vi "Log_ADAM_scan_table.vi"() -> ()   [LabVIEW 2015]
uses:
  ADAM Client/Sub VIs/ADAM Controls/Channel_State.ctl
  Anemometry/Anemometry Sub Vis/Globals/Constants_global.vi
  Anemometry/Anemometry Sub Vis/Globals/Preference_global.vi
  ADAM_Global.vi
  Anemometry/Anemometry Sub Vis/Globals/Meas_global.vi
panel:
  in  "Ventilate Lab if temp above":dbl=21.5
  in  "Averaging time (Seconds)":dbl=60.0
  out "Current time":string
  out "Started Time":string
  in  "stop":bool
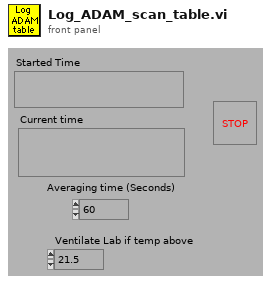
[diagram p1: front panel]
types:
  T1 = enum16{"On", "Off", "Always On", "Always Off", "Delete"}
  T2 = typedef "Channel_State.ctl" = enum16{"On", "Off", "Always On", "Always Off"}
  T3 = enum16{"Load ADAM setup from excel file", "Save ADAM setup to excel file"}
  T4 = cluster{"second":i32, "minute":i32, "hour":i32, "day of month":i32, "month":i32, "year":i32, "day of week":i32, "day of year":i32, "is DST":i32}
  T5 = typedef "Client_State_Cluster.ctl" = cluster{"Client Name":string, "Traverse level State":T6, "People to Email":string[], "Next Contact Time":dbl}
  T6 = typedef "Traverse_Level_State.ctl" = enum16{"Running", "Complete"}
  T7 = typedef "Server_Control.ctl" = cluster{"Channel Name to control":string, "Channel sharing":enum16{"Channel Unshared", "Channel Shared by Rig", "Channel Shared by Group"}, "Default Value":dbl, "Client Array":string[], "Time Stamp":timestamp, "Do Not Reset":bool}
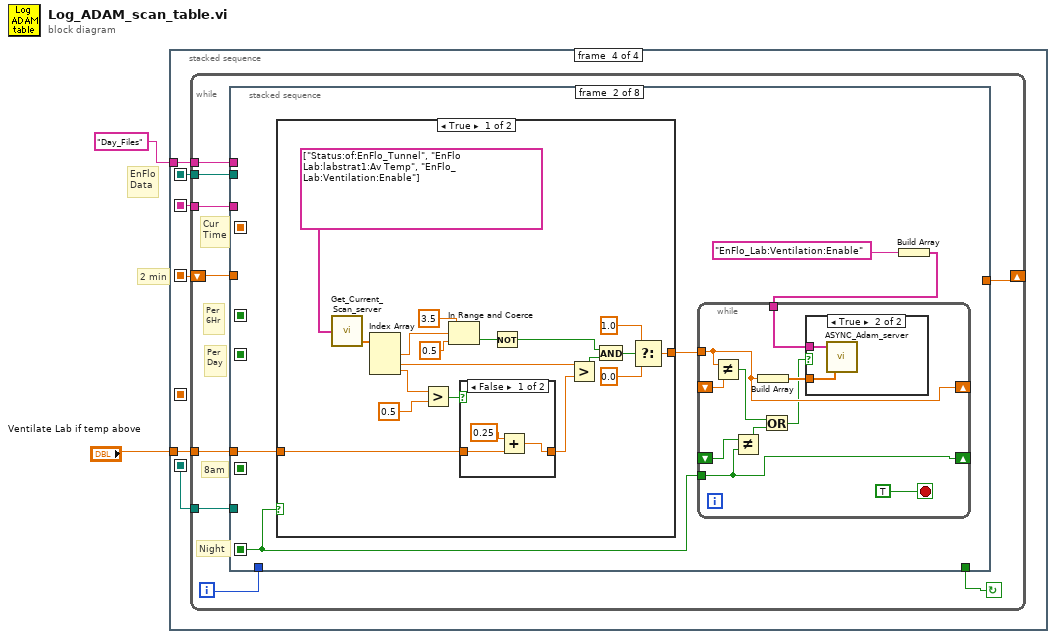
[diagram p0: block diagram]
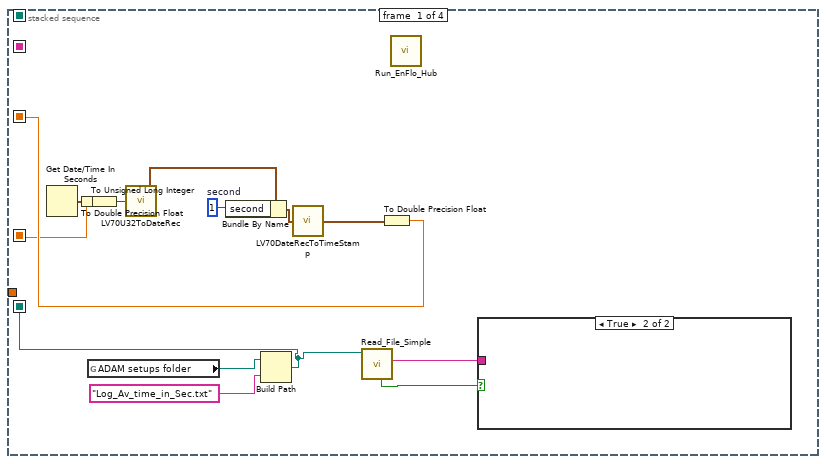
[diagram p2: hidden frame]
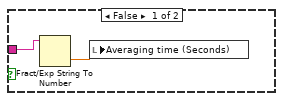
[diagram p3: hidden frame]
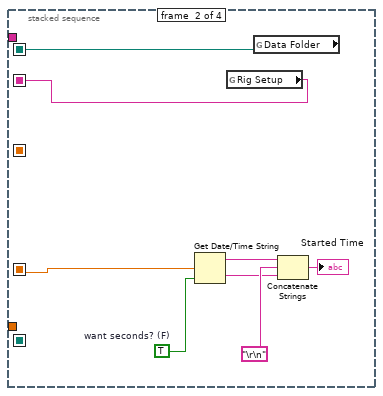
[diagram p4: hidden frame]
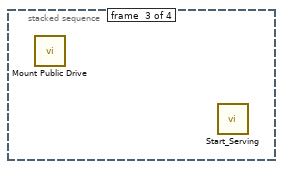
[diagram p5: hidden frame]
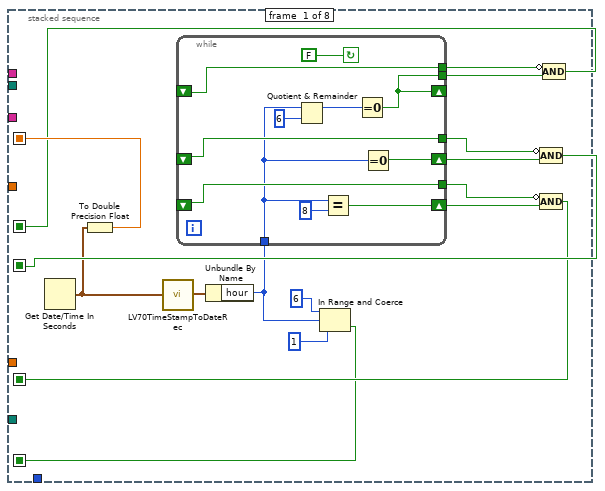
[diagram p6: hidden frame]
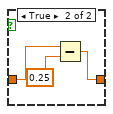
[diagram p8: hidden frame]
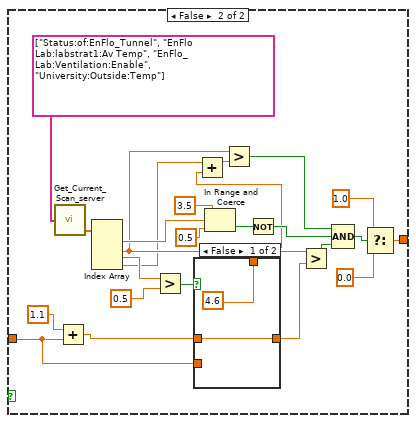
[diagram p9: hidden frame]
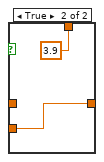
[diagram p10: hidden frame]
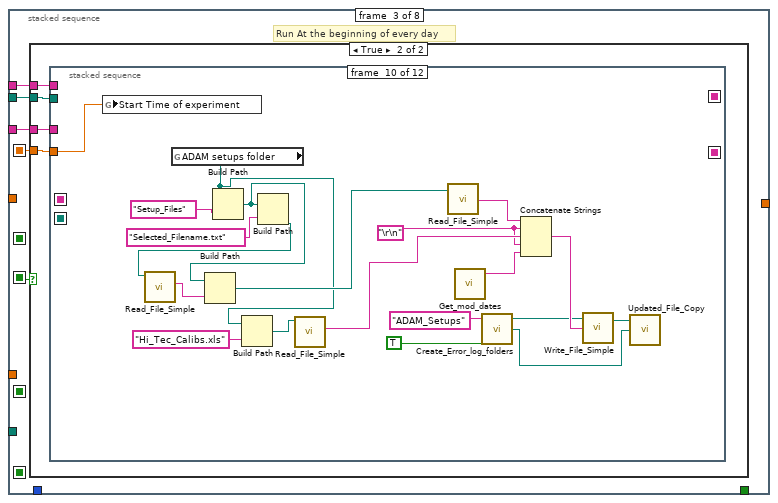
[diagram p11: hidden frame]
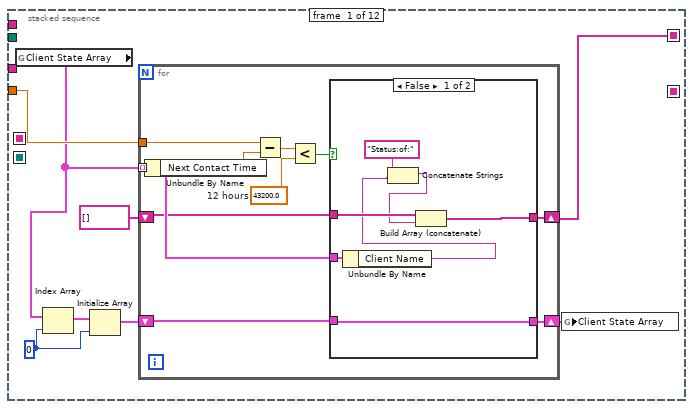
[diagram p13: hidden frame]
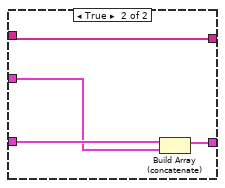
[diagram p14: hidden frame]
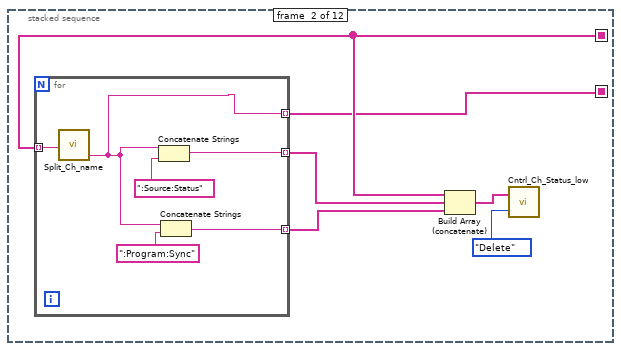
[diagram p15: hidden frame]
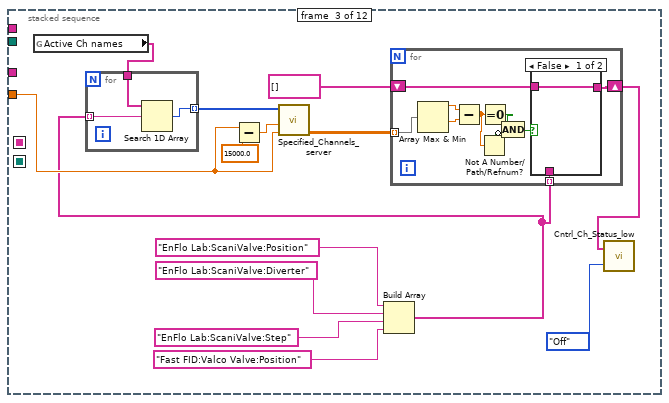
[diagram p16: hidden frame]
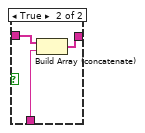
[diagram p17: hidden frame]
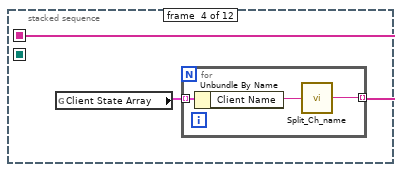
[diagram p18: hidden frame]
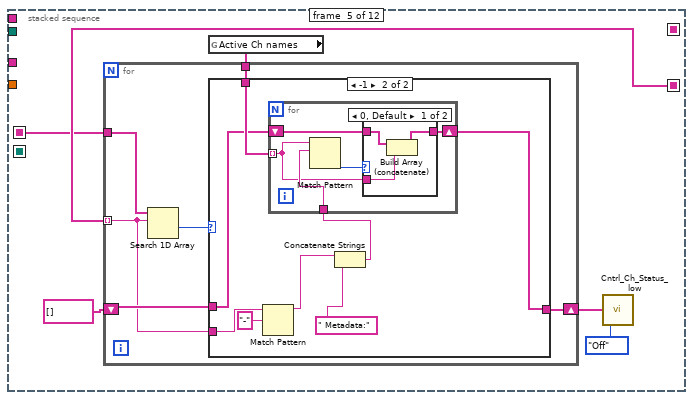
[diagram p19: hidden frame]
diagram:
  # "EnFlo\nData"
  # "2 min"
  n1 = stacked-sequence {
    seq-local: [w13 _ _ _] -> [_ _ _ w31]
    seq-local: [w12 _ _ _] -> [_ w25 _ _]
    seq-local: [_ w19 _ _] -> [_ _ _ w30]
    seq-local: [w5 _ _ _] -> [_ _ _ w28]
    seq-local: [_ w18 _ _] -> [_ _ _ w27]
    tunnel: "Day_Files" ("Input Element") -> [_ _ _ w29]
    tunnel: "Ventilate Lab if temp above" -> [_ _ _ w26]
    frame #0 {
      w15 = 1  # second
      n2 = Get Date/Time In Seconds() -> (seconds since 1Jan1904=w9:timestamp)
      n3 = To Double Precision Float(number=w9) -> (double precision float=w12:dbl)
      n4 = global read "Constants_global.vi" "ADAM setups folder"() -> (w7:path)
      n5 = To Unsigned Long Integer(number=w12) -> (unsigned 32bit integer=w11:u32)
      n6 = call <vilib>:"LV70U32ToDateRec.vi"("Time"=w11) -> ("date time rec"=w10:T4)
      n7 = Bundle By Name(cluster=w10, "second"=w15) -> (w14:T4)
      n8 = Build Path(base path=w7, name or relative path="Log_Av_time_in_Sec.txt") -> (appended path=w5:path)
      n9 = call <vilib>:"LV70DateRecToTimeStamp.vi"("date time rec"=w14) -> ("Time Stamp"=w8:timestamp)
      n10 = call "Read_File_Simple.vi"("Filename"=w5) -> ("Error?"=w3:bool, "string"=w4:string)  [unwired: 2 in, 6 out]
      n11 = To Double Precision Float(number=w8) -> (double precision float=w13:dbl)
      n12 = call "Run_EnFlo_Hub.vi"() -> ()  [unwired: 8 out]
      n13 = case shown="True" w3 {
        tunnel: w4 -> [w17 _]
        frame False {
          n14 = Fract/Exp String To Number(string=w17) -> (number=w16:dbl)  [unwired: 4 out]
          n15 = local write "Averaging time (Seconds)"(w16) -> ()
        }
        frame True {
        }
      }
    }
    frame #1 {
      w24 = TRUE  # want seconds? (F)
      n16 = Get Date/Time String(seconds (now)=w25, want seconds? (F)=w24) -> (date string=w22:string, time string=w21:string)  [unwired: 1 out]
      n17 = global read "Preference_global.vi" "Rig Setup"() -> (w18:string)
      n18 = global read "Constants_global.vi" "Data Folder"() -> (w19:path)
      n19 = Concatenate Strings(w22, "\r\n", w21) -> (→"Started Time":string)
    }
    frame #2 {
      n20 = call "Mount Public Drive.vi"() -> ()  [unwired: 12 in]
      n21 = call "Start_Serving.vi"() -> ()  [unwired: 1 out]
    }
    frame #3 {
      n22 = while {
        tunnel: w30 -> [w38]
        shift-left: w31 -> [w40]
        shift-right: [w39] -> _
        tunnel: w29 -> [w35]
        tunnel: w28 -> [w34]
        tunnel: w27 -> [w33]
        tunnel: w26 -> [w32]
        i -> [w37]
        stop <- w36 continue-if-true
        # "Night"
        # "8am"
        # "Per\n6Hr"
        # "Per\nDay"
        # "Cur\nTime"
        n23 = stacked-sequence {
          seq-local: [w49 _ _ _ _ _ _ _] -> [_ _ w141 _ _ _ _ _]
          seq-local: [w55 _ _ _ _ _ _ _] -> [_ _ w140 w367 w386 _ _ _]
          seq-local: [w52 _ _ _ _ _ _ _] -> [_ _ _ _ _ _ _ _]
          seq-local: [w45 _ _ _ _ _ _ _] -> [_ _ _ w363 _ _ _ _]
          seq-local: [w41 _ _ _ _ _ _ _] -> [_ w68 _ _ _ _ _ _]
          tunnel: [_ _ _ _ _ w388 _ _] -> w39
          tunnel: w40 -> [_ _ _ _ _ w389 _ _]
          tunnel: w38 -> [_ _ w139 w366 _ w396 _ _]
          tunnel: w37 -> [_ _ _ _ _ _ _ _]
          tunnel: [_ _ _ _ _ _ _ w428] -> w36
          tunnel: w35 -> [_ _ w138 w365 _ w397 _ _]
          tunnel: w34 -> [_ _ _ _ _ _ _ w427]
          tunnel: w33 -> [_ _ w137 w364 _ w390 _ _]
          tunnel: w32 -> [_ w69 _ _ _ _ _ _]
          frame #0 {
            n24 = Get Date/Time In Seconds() -> (seconds since 1Jan1904=w48:timestamp)
            n25 = To Double Precision Float(number=w48) -> (double precision float=w55:dbl)
            n26 = call <vilib>:"LV70TimeStampToDateRec.vi"("time stamp"=w48) -> ("date time rec"=w56:T4)
            n27 = Unbundle By Name(w56) -> ("hour"=w44:i32)
            n28 = while {
              tunnel: [w62] -> w50
              shift-left: _ -> [w62]
              shift-right: [w63] -> w51
              tunnel: [w64] -> w53
              tunnel: [w65] -> w54
              tunnel: w44 -> [w59]
              shift-left: _ -> [w64]
              shift-right: [w65] -> _
              tunnel: [w60] -> w47
              shift-right: [w57] -> w46
              shift-left: _ -> [w60]
              stop <- FALSE continue-if-true
              n29 = Quotient & Remainder(x=w59, y=6) -> (x-y*floor(x/y)=w66:i32)  [unwired: 1 out]
              n30 = Equal?(x=w59, y=8) -> (x = y?=w57:bool)
              n31 = Equal To 0?(x=w66) -> (x = 0?=w65:bool)
              n32 = Equal To 0?(x=w59) -> (x = 0?=w63:bool)
            }
            n33 = In Range and Coerce(upper limit=6, x=w44, lower limit=1) -> (In Range?=w41:bool)  [unwired: 1 out]
            n34 = Compound Arithmetic op=AND(invert w50, w51) -> (w49:bool)
            n35 = Compound Arithmetic op=AND(invert w47, w46) -> (w45:bool)
            n36 = Compound Arithmetic op=AND(invert w53, w54) -> (w52:bool)
          }
          frame #1 {
            n37 = case shown="True" w68 {
              tunnel: [w95 w126] -> w70
              tunnel: w69 -> [w85 w109]
              frame True {
                n38 = call "Get_Current_Scan_server.vi"("Desired Channels"=string[] ["Status:of:EnFlo_Tunnel", "EnFlo Lab:labstrat1:Av Temp", "EnFlo_Lab:Ventilation:Enable"]) -> ("Numerical Values"=w101:dbl[])  [unwired: 2 out]
                n39 = Index Array(array=w101) -> (element #1=w94:dbl, element #2=w100:dbl, element #3=w89:dbl)  [unwired: 3 in]
                n40 = Greater?(x=w89, y=0.5) -> (0:w87:bool)
                n41 = In Range and Coerce(upper limit=3.5, x=w94, lower limit=0.5) -> (In Range?=w91:bool)  [unwired: 1 out]
                n42 = case shown="False" w87 {
                  tunnel: [w104 w106] -> w86
                  tunnel: w85 -> [w105 w108]
                  frame False {
                    n43 = Add(x=0.25, y=w105) -> (x+y=w104:dbl)
                  }
                  frame True {
                    n44 = Subtract(x=w108, y=0.25) -> (x-y=w106:dbl)
                  }
                }
                n45 = Not(x=w91) -> (.not. x?=w90:bool)
                n46 = Greater?(x=w100, y=w86) -> (0:w99:bool)
                n47 = And(x=w90, y=w99) -> (x .and. y?=w98:bool)
                n48 = Select(t=1.0, s=w98, f=0.0) -> (s? t:f=w95:dbl)
              }
              frame False {
                n49 = call "Get_Current_Scan_server.vi"("Desired Channels"=string[] ["Status:of:EnFlo_Tunnel", "EnFlo Lab:labstrat1:Av Temp", "EnFlo_Lab:Ventilation:Enable", "University:Outside:Temp"]) -> ("Numerical Values"=w131:dbl[])  [unwired: 2 out]
                n50 = Add(x=1.1, y=w109) -> (x+y=w116:dbl)
                n51 = Index Array(array=w131) -> (element #1=w125:dbl, element #2=w114:dbl, element #3=w120:dbl, element #4=w113:dbl)  [unwired: 4 in]
                n52 = Greater?(x=w120, y=0.5) -> (0:w118:bool)
                n53 = case shown="False" w118 {
                  tunnel: [w134 w135] -> w117
                  tunnel: w116 -> [w134 _]
                  tunnel: [4.6 ("y") 3.9 ("y")] -> w110
                  tunnel: w109 -> [_ w135]
                  frame False {
                  }
                  frame True {
                  }
                }
                n54 = Add(x=w113, y=w110) -> (x+y=w112:dbl)
                n55 = In Range and Coerce(upper limit=3.5, x=w125, lower limit=0.5) -> (In Range?=w122:bool)  [unwired: 1 out]
                n56 = Greater?(x=w114, y=w112) -> (0:w111:bool)
                n57 = Not(x=w122) -> (.not. x?=w121:bool)
                n58 = Greater?(x=w114, y=w117) -> (0:w130:bool)
                n59 = Compound Arithmetic op=AND(w111, w121, w130) -> (w129:bool)
                n60 = Select(t=1.0, s=w129, f=0.0) -> (s? t:f=w126:dbl)
              }
            }
            n61 = Build Array("EnFlo_Lab:Ventilation:Enable") -> (w71:string[])
            n62 = while {
              shift-right: [w80] -> _
              shift-left: _ -> [w81]
              tunnel: w70 -> [w80]
              tunnel: w71 -> [w78]
              shift-right: [w77] -> _
              shift-left: _ -> [w76]
              tunnel: w68 -> [w77]
              stop <- TRUE stop-if-true
              n63 = Not Equal?(x=w80, y=w81) -> (x != y?=w74:bool)
              n64 = Not Equal?(x=w76, y=w77) -> (x != y?=w75:bool)
              n65 = Build Array(w80) -> (w82:dbl[])
              n66 = Or(x=w74, y=w75) -> (x .or. y?=w73:bool)
              n67 = case shown="True" w73 {
                tunnel: w82 -> [_ w84]
                tunnel: w78 -> [_ w83]
                frame False {
                }
                frame True {
                  n68 = call "ASYNC_Adam_server.vi"("Values"=w84, "Channel Names"=w83) -> ()  [unwired: 1 in, 3 out]
                }
              }
            }
          }
          frame #2 {
            # "Run At the beginning of every day"
            n69 = case shown="True" w141 {
              tunnel: w140 -> [_ w145]
              tunnel: w139 -> [_ w144]
              tunnel: w138 -> [_ w143]
              tunnel: w137 -> [_ w142]
              frame False {
              }
              frame True {
                n70 = stacked-sequence {
                  seq-local: [w146 _ _ _ _ _ _ _ _ _ _ _] -> [_ w180 _ _ _ _ _ _ w300 _ _ _]
                  seq-local: [_ w176 _ _ _ _ _ _ _ _ _ _] -> [_ _ _ _ w228 _ _ _ _ _ _ _]
                  seq-local: [_ _ _ w218 _ _ _ _ _ _ _ _] -> [_ _ _ _ w225 _ _ _ _ _ _ _]
                  seq-local: [_ _ _ _ _ _ _ _ _ _ w349 _] -> [_ _ _ _ _ _ _ _ _ _ _ w353]
                  tunnel: w145 -> [w153 _ w197 _ _ _ _ _ _ w347 _ w354]
                  tunnel: w144 -> [_ _ _ _ _ _ _ _ _ _ _ _]
                  tunnel: w143 -> [_ _ _ _ _ _ _ _ _ _ _ _]
                  tunnel: w142 -> [_ _ _ _ _ _ _ _ _ _ _ _]
                  frame #0 {
                    w151 = 0 ("Index")
                    n71 = global read "ADAM_Global.vi" "Client State Array"() -> (w152:T5[])
                    n72 = Index Array(array=w152, index=w151) -> (element=w150:T5)
                    n73 = Initialize Array(w150, w151) -> (w149:T5[])
                    n74 = for {
                      tunnel: w152 -> [w156] mode=indexing
                      shift-right: [w157] -> w148
                      shift-left: w149 -> [w158]
                      tunnel: w153 -> [w163]
                      shift-right: [w154] -> w146
                      shift-left: string[] [] -> [w155]
                      w160 = 43200.0  # 12 hours
                      n75 = Unbundle By Name(w156) -> ("Next Contact Time"=w162:dbl)
                      n76 = Subtract(x=w163, y=w162) -> (x-y=w161:dbl)
                      n77 = Less?(x=w161, y=w160) -> (x < y?=w159:bool)
                      n78 = case shown="False" w159 {
                        tunnel: w158 -> [w170 w174]
                        tunnel: [w170 w173] -> w157
                        tunnel: w156 -> [w169 w172]
                        tunnel: w155 -> [w168 w171]
                        tunnel: [w167 w171] -> w154
                        frame False {
                          n79 = Unbundle By Name(w169) -> ("Client Name"=w165:string)
                          n80 = Concatenate Strings("Status:of:", w165) -> (w164:string)
                          n81 = Build Array (concatenate)(w168, w164) -> (w167:string[])
                        }
                        frame True {
                          n82 = Build Array (concatenate)(w174, w172) -> (w173:T5[])
                        }
                      }
                    }
                    n83 = global write "ADAM_Global.vi" "Client State Array"(w148) -> ()
                  }
                  frame #1 {
                    n84 = for {
                      tunnel: w180 -> [w186] mode=indexing
                      tunnel: [w183] -> w178 mode=indexing
                      tunnel: [w182] -> w177 mode=indexing
                      tunnel: [w181] -> w176 mode=indexing
                      n85 = call "Split_Ch_name.vi"("Ch name"=w186) -> ("Low level"=w181:string)  [unwired: 2 out]
                      n86 = Concatenate Strings(w181, ":Source:Status") -> (w183:string)
                      n87 = Concatenate Strings(w181, ":Program:Sync") -> (w182:string)
                    }
                    n88 = Build Array (concatenate)(w180, w178, w177) -> (w179:string[])
                    n89 = call "Cntrl_Ch_Status_low.vi"("Mode"=T1."Delete", "Channel names"=w179) -> ()  [unwired: 1 out]
                  }
                  frame #2 {
                    n90 = global read "ADAM_Global.vi" "Active Ch names"() -> (w200:string[])
                    n91 = Subtract(x=w197, y=15000.0) -> (x-y=w195:dbl)
                    n92 = Build Array("EnFlo Lab:ScaniValve:Position", "EnFlo Lab:ScaniValve:Diverter", "EnFlo Lab:ScaniValve:Step", "Fast FID:Valco Valve:Position") -> (w193:string[])
                    n93 = for {
                      tunnel: w200 -> [w217]
                      tunnel: w193 -> [w216] mode=indexing
                      tunnel: [w215] -> w198 mode=indexing
                      n94 = Search 1D Array(1D array=w217, element=w216) -> (index of element=w215:i32)  [unwired: 1 out]
                    }
                    n95 = call "Specified_Channels_server.vi"("End time"=w197, "Start time"=w195, "Requested channels"=w198) -> ("Output array"=w194:dbl[][])  [unwired: 2 in, 4 out]
                    n96 = for {
                      tunnel: w194 -> [w207] mode=indexing
                      shift-right: [w208] -> w188
                      shift-left: string[] [] -> [w202]
                      tunnel: w193 -> [w203] mode=indexing
                      n97 = Array Max & Min(array=w207) -> (max value=w210:dbl, min value=w209:dbl)  [unwired: 2 out]
                      n98 = Subtract(x=w210, y=w209) -> (x-y=w206:dbl)
                      n99 = Not A Number/Path/Refnum?(number/path/refnum=w206) -> (NaN/Path/Refnum?=w204:bool)
                      n100 = Equal To 0?(x=w206) -> (x = 0?=w201:bool)
                      n101 = Compound Arithmetic op=AND(w201, invert w204) -> (w205:bool)
                      n102 = case shown="False" w205 {
                        tunnel: [w211 w214] -> w208
                        tunnel: w203 -> [_ w213]
                        tunnel: w202 -> [w211 w212]
                        frame False {
                        }
                        frame True {
                          n103 = Build Array (concatenate)(w212, w213) -> (w214:string[])
                        }
                      }
                    }
                    n104 = call "Cntrl_Ch_Status_low.vi"("Mode"=T1."Off", "Channel names"=w188) -> ()  [unwired: 1 out]
                  }
                  frame #3 {
                    n105 = global read "ADAM_Global.vi" "Client State Array"() -> (w219:T5[])
                    n106 = for {
                      tunnel: w219 -> [w222] mode=indexing
                      tunnel: [w220] -> w218 mode=indexing
                      n107 = Unbundle By Name(w222) -> ("Client Name"=w221:string)
                      n108 = call "Split_Ch_name.vi"("Ch name"=w221) -> ("Middle"=w220:string)  [unwired: 2 out]
                    }
                  }
                  frame #4 {
                    n109 = global read "ADAM_Global.vi" "Active Ch names"() -> (w226:string[])
                    n110 = for {
                      tunnel: w228 -> [w229] mode=indexing
                      shift-right: [w232] -> w224
                      shift-left: string[] [] -> [w233]
                      tunnel: w226 -> [w231]
                      tunnel: w225 -> [w230]
                      n111 = Search 1D Array(1D array=w230, element=w229) -> (index of element=w234:i32)  [unwired: 1 out]
                      n112 = case shown="-1" w234 {
                        tunnel: w233 -> [w235 w241]
                        tunnel: [w235 w240] -> w232
                        tunnel: w229 -> [_ w236]
                        tunnel: w231 -> [_ w242]
                        frame 0, Default {
                        }
                        frame -1 {
                          n113 = Match Pattern(string=w236, regular expression="-") -> (before substring=w237:string)  [unwired: 4 out]
                          n114 = Concatenate Strings(w237, " Metadata:" ("Substring")) -> (w239:string)
                          n115 = for {
                            shift-right: [w246] -> w240
                            shift-left: w241 -> [w247]
                            tunnel: w239 -> [w245]
                            tunnel: w242 -> [w244] mode=indexing
                            n116 = Match Pattern(string=w244, regular expression=w245) -> (offset past match=w248:i32)  [unwired: 4 out]
                            n117 = case shown="0, Default" w248 {
                              tunnel: w247 -> [w250 w252]
                              tunnel: [w249 w252] -> w246
                              tunnel: w244 -> [w251 _]
                              frame 0, Default {
                                n118 = Build Array (concatenate)(w250, w251) -> (w249:string[])
                              }
                              frame -1 {
                              }
                            }
                          }
                        }
                      }
                    }
                    n119 = call "Cntrl_Ch_Status_low.vi"("Mode"=T1."Off", "Channel names"=w224) -> ()  [unwired: 1 out]
                  }
                  frame #5 {
                    n120 = Build Array("EnFlo_Tunnel:Heater:Enable") -> (w258:string[])
                    n121 = call "Get_Current_Scan_server.vi"("Desired Channels"=w258) -> ("Numerical Values"=w257:dbl[])  [unwired: 2 out]
                    n122 = Index Array(array=w257, index=0) -> (element=w255:dbl)
                    n123 = Less?(x=w255, y=0.5) -> (x < y?=w253:bool)
                    n124 = case shown="True" w253 {
                      frame False {
                      }
                      frame True {
                        w264 = "EnFlo_Tunnel:Setpo"
                        n125 = global read "ADAM_Global.vi" "Active Ch names"() -> (w262:string[])
                        n126 = String Length(string=w264) -> (length=w263:i32)
                        n127 = for {
                          shift-right: [w272] -> w261
                          shift-left: string[] [] -> [w274]
                          tunnel: w262 -> [w273] mode=indexing
                          tunnel: w263 -> [w276]
                          tunnel: w264 -> [w275]
                          tunnel: "EnFlo_Tunnel:Power" -> [w270]
                          n128 = String Subset(string=w273, length (rest)=w276) -> (substring=w271:string)  [unwired: 1 out]
                          n129 = Equal?(x=w271, y=w275) -> (x = y?=w268:bool)
                          n130 = Equal?(x=w271, y=w270) -> (x = y?=w269:bool)
                          n131 = Or(x=w268, y=w269) -> (x .or. y?=w267:bool)
                          n132 = case shown="True" w267 {
                            tunnel: w274 -> [w277 w280]
                            tunnel: w273 -> [_ w279]
                            tunnel: [w277 w278] -> w272
                            frame False {
                            }
                            frame True {
                              n133 = Build Array (concatenate)(w280, w279) -> (w278:string[])
                            }
                          }
                        }
                        n134 = call "Adam_Ch_on_off.vi"("Ch State"=Channel_State."Off", "ADAM Ch Names"=w261) -> ()  [unwired: 1 out]
                      }
                    }
                  }
                  frame #6 {
                    n135 = call "Read_Write_ADAM_setup.vi"("Mode"=T3."Save ADAM setup to excel file") -> ()  [unwired: 4 out]
                  }
                  frame #7 {
                    w285 = 5400.0  # 1.5 Hrs in seconds
                    n136 = Build Array("GMU:Source:Meas Q", "GMU:Source:Est Time") -> (w292:string[])
                    n137 = call "Get_Current_Scan_server.vi"("Desired Channels"=w292) -> ("Numerical Values"=w287:dbl[])  [unwired: 2 out]
                    n138 = Index Array(array=w287, index=0 ("Index")) -> (element=w289:dbl)
                    n139 = Index Array(array=w287, index=1 ("Index")) -> (element=w286:dbl)
                    n140 = Less?(x=w289, y=0.01) -> (x < y?=w283:bool)
                    n141 = Greater?(x=w286, y=w285) -> (0:w284:bool)
                    n142 = And(x=w283, y=w284) -> (x .and. y?=w282:bool)
                    n143 = case shown="True" w282 {
                      frame False {
                      }
                      frame True {
                        w295 = FALSE  # Activate channels
                        w296 = enum16{"Channel Name", "Main Address"}."Channel Name" ("Control on")
                        n144 = call "Ch_Active_Control.vi"("Match"="GMU:", "Activate Channels?"=w295, "Control on"=w296) -> ()  [unwired: 1 in, 2 out]
                        n145 = call "Ch_Active_Control.vi"("Match"="source", "Activate Channels?"=w295, "Control on"=w296) -> ()  [unwired: 1 in, 2 out]
                      }
                    }
                  }
                  frame #8 {
                    w304 = 0 ("Index")
                    n146 = global read "ADAM_Global.vi" "Server Control Array"() -> (w301:T7[])
                    n147 = Index Array(array=w301, index=w304) -> (element=w303:T7)
                    n148 = Initialize Array(w303, w304) -> (w302:T7[])
                    n149 = for {
                      tunnel: w301 -> [w306] mode=indexing
                      shift-right: [w311] -> w299
                      shift-left: w302 -> [w312]
                      tunnel: w300 -> [w310]
                      n150 = Unbundle By Name(w306) -> ("Client Array"=w309:string[])
                      n151 = for {
                        tunnel: w310 -> [w317]
                        tunnel: w309 -> [w315] mode=indexing
                        shift-right: [w313] -> w305
                        shift-left: string[] [] -> [w314]
                        n152 = Search 1D Array(1D array=w317, element=w315) -> (index of element=w316:i32)  [unwired: 1 out]
                        n153 = case shown="0, Default" w316 {
                          tunnel: w315 -> [_ w321]
                          tunnel: w314 -> [w318 w320]
                          tunnel: [w318 w319] -> w313
                          frame 0, Default {
                          }
                          frame -1 {
                            n154 = Build Array (concatenate)(w320, w321) -> (w319:string[])
                          }
                        }
                      }
                      n155 = Array Size(array=w305) -> (size(s)=w307:i32)
                      n156 = case shown="0" w307 {
                        tunnel: w312 -> [w322 w326]
                        tunnel: [w322 w327] -> w311
                        tunnel: w306 -> [_ w325]
                        tunnel: w305 -> [_ w324]
                        frame 0 {
                        }
                        frame 1, Default {
                          n157 = Bundle By Name(cluster=w325, "Client Array"=w324) -> (w323:T7)
                          n158 = Build Array (concatenate)(w326, w323) -> (w327:T7[])
                        }
                      }
                    }
                    n159 = global write "ADAM_Global.vi" "Server Control Array"(w299) -> ()
                  }
                  frame #9 {
                    w335 = "\r\n"
                    n160 = global write "Meas_global.vi" "Start Time of experiment"(w347) -> ()
                    n161 = global read "Constants_global.vi" "ADAM setups folder"() -> (w338:path)
                    n162 = Build Path(base path=w338, name or relative path="Setup_Files") -> (appended path=w342:path)
                    n163 = Build Path(base path=w338, name or relative path="Hi_Tec_Calibs.xls") -> (appended path=w337:path)
                    n164 = Build Path(base path=w342, name or relative path="Selected_Filename.txt" ("Substring")) -> (appended path=w344:path)
                    n165 = call "Read_File_Simple.vi"("Filename"=w344) -> ("string"=w343:string)  [unwired: 2 in, 7 out]
                    n166 = Build Path(base path=w342, name or relative path=w343) -> (appended path=w341:path)
                    n167 = call "Read_File_Simple.vi"("Filename"=w337) -> ("string"=w336:string)  [unwired: 2 in, 7 out]
                    n168 = call "Read_File_Simple.vi"("Filename"=w341) -> ("string"=w340:string)  [unwired: 2 in, 7 out]
                    n169 = call "Get_mod_dates.vi"() -> ("Output string"=w334:string)  [unwired: 1 in, 4 out]
                    n170 = call "Create_Error_log_folders.vi"("Per Day Log File?"=TRUE, "Log Filename"="ADAM_Setups" ("Substring")) -> ("Server copy Location"=w328:path, "Local Log File"=w330:path)  [unwired: 1 in, 1 out]
                    n171 = Concatenate Strings(w340, w335, w336, w335, w334) -> (w331:string)
                    n172 = call "Write_File_Simple.vi"("character string"=w331, "file path"=w330) -> ("file path Out"=w329:path)  [unwired: 1 in, 1 out]
                    n173 = call "Updated_File_Copy.vi"("Target Path"=w328, "Source Path"=w329) -> ()  [unwired: 2 out]
                  }
                  frame #10 {
                    n174 = global read "Constants_global.vi" "Data Folder Local"() -> (w350:path)
                    n175 = Build Path(base path=w350, name or relative path="Results_Summary_files") -> (appended path=w349:path)
                  }
                  frame #11 {
                    # "If the summary files are more than 60 days old delete them"
                    n176 = To Unsigned Long Integer(number=w354) -> (unsigned 32bit integer=w351:u32)
                    n177 = call "Get_folder_and_filenames.vi"("file path (dialog if empty)"=w353) -> ("Files"=w352:path[])  [unwired: 1 out]
                    n178 = for {
                      tunnel: w352 -> [w356] mode=indexing
                      tunnel: w351 -> [w361]
                      # "60 days in seconds"
                      n179 = File/Directory Info(path=w356) -> (last mod=w355:timestamp)  [unwired: 1 in, 6 out]
                      n180 = To Unsigned Long Integer(number=w355) -> (unsigned 32bit integer=w360:u32)
                      n181 = Subtract(x=w361, y=w360) -> (x-y=w359:u32)
                      n182 = Greater?(x=w359, y=u32 5184000) -> (0:w357:bool)
                      n183 = case shown="False" w357 {
                        tunnel: w356 -> [_ w362]
                        frame False {
                        }
                        frame True {
                          n184 = Delete(path (use dialog)=w362) -> ()  [unwired: 1 in, 6 out]
                        }
                      }
                    }
                  }
                }
              }
            }
          }
          frame #3 {
            # "At 8am every day"
            n185 = case shown="True" w363 {
              tunnel: w367 -> [_ w371]
              tunnel: w366 -> [_ w370]
              tunnel: w365 -> [_ w369]
              tunnel: w364 -> [_ w368]
              frame False {
              }
              frame True {
                n186 = stacked-sequence {
                  seq-local: [w379 _] -> [_ w385]
                  tunnel: w371 -> [w383 _]
                  tunnel: w370 -> [w372 _]
                  tunnel: w369 -> [w377 _]
                  tunnel: w368 -> [w373 _]
                  frame #0 {
                    n187 = Subtract(x=w383, y=36000.0) -> (x-y=w381:dbl)
                    n188 = call "Sec_to_date_filename.vi"("seconds"=w381) -> ("Year"=w378:string, "Month"=w382:string, "Day"=w375:string)  [unwired: 1 out]
                    n189 = Concatenate Strings(w375, ".xls" ("string")) -> (w374:string)
                    n190 = Build Array(w378, w373, w377, w382, w374) -> (w380:string[])
                    n191 = call "Build_Pathname.vi"("PathElements"=w380, "PathnameIn"=w372) -> ("AppendedPath"=w379:path)
                  }
                  frame #1 {
                    # "This VI emails a summary of all the server errors that occured Yesterday"
                    n192 = call "Adam_server_messages.vi"("Filename"=w385) -> ()  [unwired: 1 out]
                  }
                }
              }
            }
          }
          frame #4 {
            n193 = call "EnFlo_Seeder_Control.vi"("Current Time (s)"=w386) -> ()
            n194 = Wait (ms)(milliseconds to wait=u32 1000 ("milliseconds to Wait")) -> ()  [unwired: 1 out]
          }
          frame #5 {
            n195 = Divide(x="Averaging time (Seconds)", y=60.0) -> (x/y=w394:dbl)
            n196 = Divide(x="Averaging time (Seconds)", y=2.0) -> (x/y=w391:dbl)
            n197 = Add(x=w391, y=w389) -> (x+y=w407:dbl)
            n198 = call "Sec_to_date_filename.vi"("seconds"=w407) -> ("Year"=w402:string, "Month"=w403:string, "Day"=w398:string)  [unwired: 1 out]
            n199 = Concatenate Strings(w398, ".xls" ("string")) -> (w400:string)
            n200 = Build Array(w402, w390, w397, w403, w400) -> (w401:string[])
            n201 = call "Time_elapsed.vi"("End of previous average in"=w389, "Averaging time (mins)"=w394) -> ("End of previous average out"=w388:dbl, "End of period"=w405:dbl, "Start of period"=w406:dbl, "Time elapsed ?"=w404:bool)  [unwired: 2 in]
            n202 = case shown="True" w404 {
              tunnel: w405 -> [_ w410]
              tunnel: w406 -> [_ w411]
              tunnel: w396 -> [_ w409]
              tunnel: w401 -> [_ w408]
              frame False {
              }
              frame True {
                n203 = stacked-sequence {
                  tunnel: w411 -> [w420 _]
                  tunnel: w410 -> [w419 _]
                  tunnel: w409 -> [w412 _]
                  tunnel: w408 -> [w415 _]
                  frame #0 {
                    n204 = global read "ADAM_Global.vi" "2 Min average comment"() -> (w418:string)
                    n205 = global read "Meas_global.vi" "Error Messages"() -> (w417:string)
                    n206 = call "Build_Pathname.vi"("PathElements"=w415, "PathnameIn"=w412) -> ("AppendedPath"=w414:path)
                    n207 = call "Create_directory_path.vi"("Path name"=w414) -> ("Path name Out"=w413:path)  [unwired: 1 in, 1 out]
                    n208 = Concatenate Strings(w418, w417) -> (w416:string)
                    n209 = call "Write_to_log_file.vi"("User added comment"=w416, "End time"=w419, "Start time"=w420, "Folder/file"=w413) -> ()  [unwired: 5 in, 3 out]
                  }
                  frame #1 {
                    w421 = ""
                    n210 = global write "ADAM_Global.vi" "2 Min average comment"(w421) -> ()
                    n211 = global write "Meas_global.vi" "Error Messages"(w421) -> ()
                  }
                }
              }
            }
          }
          frame #6 {
            w426 = TRUE  # want seconds? (F)
            n212 = Get Date/Time String(want seconds? (F)=w426) -> (date string=w424:string, time string=w423:string)  [unwired: 2 out]
            n213 = Concatenate Strings(w424, "\r\n", w423) -> (→"Current time":string)
          }
          frame #7 {
            n214 = while {
              shift-right: [w430] -> _
              shift-left: _ -> [w434]
              tunnel: w427 -> [w431]
              stop <- TRUE stop-if-true
              n215 = local read "Averaging time (Seconds)"() -> (w430:dbl)
              n216 = Not Equal?(x=w430, y=w434) -> (x != y?=w432:bool)
              n217 = case shown="True" w432 {
                tunnel: w431 -> [_ w435]
                tunnel: w430 -> [_ w437]
                frame False {
                }
                frame True {
                  n218 = Number To Fractional String(number=w437, precision (6)=i16 6) -> (F-format string=w436:string)  [unwired: 2 out]
                  n219 = call "Write_File_Simple.vi"("character string"=w436, "file path"=w435) -> ()  [unwired: 1 in, 2 out]
                }
              }
            }
            n220 = Not(x="stop") -> (.not. x?=w428:bool)
          }
        }
      }
    }
  }
